vi "WT300 Get Current.vi"(8 "error in (no error)":errorcluster, 10 "Update Rate (500m s)":dbl(ring)=0.5 format="%#_2f" items=["100m"=0.1, "250m"=0.25, "500m"=0.5, "1"=1.0, "2"=2.0, "5"=5.0], 11 "VISA Refnum in":refnum<visa-resource-name>) -> (0 "error out":errorcluster, 1 "Function":string[](array[string]), 2 "Measurement":dbl[](array[numeric]), 3 "VISA Refnum out":refnum<visa-resource-name>)   [LabVIEW 2016]
uses:
  Public/Utility/Function/Create Function String (Current).vi
  Public/Data/Read Measurement (Normal).vi
  Yokogawa WT300 Series.lvlib
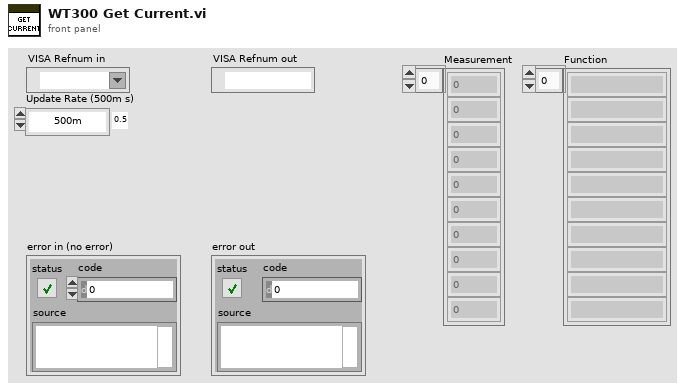
[diagram p1: front panel]
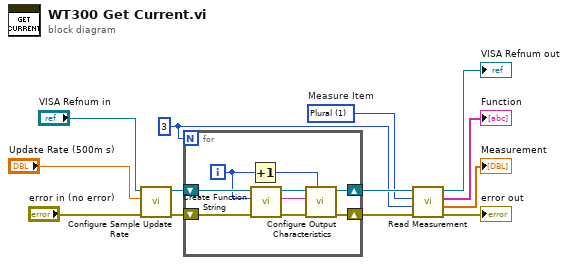
[diagram p0: block diagram]
diagram:
  w6 = 3
  w7 = 1 items=["One", "Plural"]  # Measure Item
  n1 = call "Configure Sample Update Rate.vi"("error in (no error)"="error in (no error)", "Update Rate (500m s)"="Update Rate (500m s)", "VISA resource name"="VISA Refnum in") -> ("error out"=w4:errorcluster, "VISA resource name out"=w2:refnum<visa-resource-name>)  [unwired: 7 in]
  n2 = for {
    N: w6 -> [_]
    shift-right: [w19] -> w9
    shift-left: w2 -> [w21]
    shift-right: [w18] -> w8
    shift-left: w4 -> [w20]
    i -> [w14]
    n3 = Increment(x=w14) -> (x+1=w15:i32)
    n4 = call-poly "Create Function String.vi"("error in (no error)"=w20, "Function (0: I)"=w14, "VISA resource name"=w21) -> ("error out"=w16:errorcluster, "Function String"=w22:string, "VISA resource name out"=w17:refnum<visa-resource-name>)  [unwired: 6 in]
    n5 = call "Configure Output Characteristics.vi"("Item (1)"=w15, "error in (no error)"=w16, "Function (Empty)"=w22, "VISA resource name"=w17) -> ("error out"=w18:errorcluster, "VISA resource name out"=w19:refnum<visa-resource-name>)  [unwired: 6 in]
  }
  n6 = call-poly "Read Measurement.vi"("error in (no error)"=w8, "Number of Item (15)"=w6, "Measure Item (1: Plural)"=w7, "VISA resource name"=w9) -> ("error out"=→"error out":errorcluster, "Measurement"=→"Measurement":dbl[], "Function"=→"Function":string[], "VISA resource name out"=→"VISA Refnum out":refnum<visa-resource-name>)  [unwired: 4 in]
